vi "Assignment 1.vi"() -> ()   [LabVIEW 2024]
panel:
  out "t Result":dbl
  in  "Value 2":dbl
  in  "Value 1":dbl
  out "Perimeter  Result (m)":dbl
  out "Area Result (m^2)":dbl
  in  "Length (m)":dbl
  in  "Width (m)":dbl
  out "Multiply Result":dbl
  in  "Interger  4":dbl
  in  "Interger  3":dbl
  in  "Interger  2":dbl
  in  "Interger 1":dbl
  out "Add Results":dbl
  # "Problem 1: Adding/Multiplying Intergers"
  # "Problem 2: Area/Perimeter of rectangle"
  # "A=bh/ A=WL"
  # "Problem 3: Value Equation"
  # "Solve V(t)=-2200t + 24000; t=7."
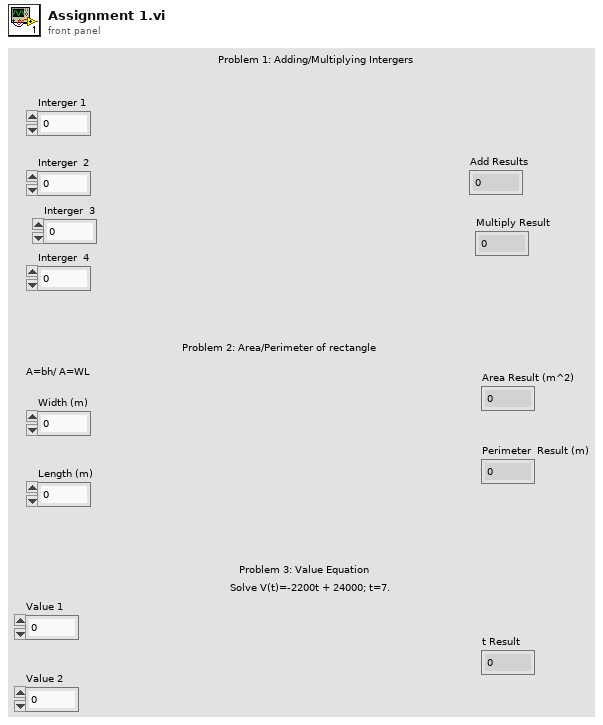
[diagram p1: front panel]
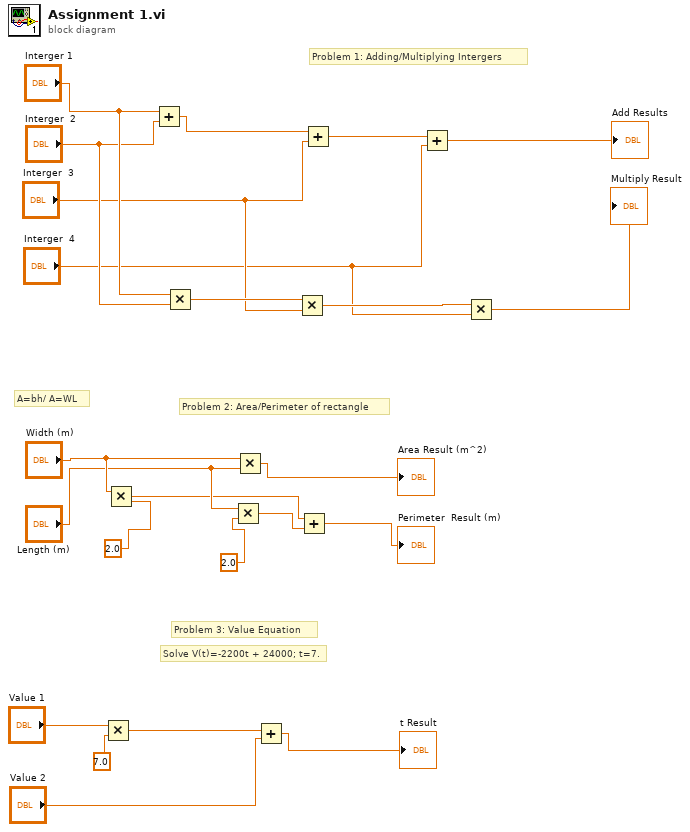
[diagram p0: block diagram]
diagram:
  # "Solve V(t)=-2200t + 24000; t=7."
  # "Problem 3: Value Equation"
  # "A=bh/ A=WL"
  # "Problem 2: Area/Perimeter of rectangle"
  # "Problem 1: Adding/Multiplying Intergers"
  n1 = Multiply(x="Value 1", y=7.0) -> (x*y=w2:dbl)
  n2 = Multiply(x="Width (m)", y=2.0) -> (x*y=w8:dbl)
  n3 = Add(x="Interger 1", y="Interger  2") -> (x+y=w23:dbl)
  n4 = Multiply(x="Interger 1", y="Interger  2") -> (x*y=w17:dbl)
  n5 = Multiply(x="Length (m)", y=2.0) -> (x*y=w7:dbl)
  n6 = Multiply(x="Width (m)", y="Length (m)") -> (x*y=→"Area Result (m^2)":dbl)
  n7 = Add(x=w2, y="Value 2") -> (x+y=→"t Result":dbl)
  n8 = Multiply(x=w17, y="Interger  3") -> (x*y=w15:dbl)
  n9 = Add(x=w8, y=w7) -> (x+y=→"Perimeter  Result (m)":dbl)
  n10 = Add(x=w23, y="Interger  3") -> (x+y=w22:dbl)
  n11 = Add(x=w22, y="Interger  4") -> (x+y=→"Add Results":dbl)
  n12 = Multiply(x=w15, y="Interger  4") -> (x*y=→"Multiply Result":dbl)
